vi "FTW-Actor-LocalMessage-Send.vi"(0 "FTW-ActorInstance In":refnum<class "FTW-ActorInstance.lvclass">, 5 "Message Header":string, 7 "Message Body":string, 11 "error in":errorcluster) -> (15 "error out":errorcluster)   [LabVIEW 2013, in "FTW-ActorInstance.lvclass"]
uses:
  FTW-ActorInstance.lvclass
  Message/Base/FTW-Message.lvclass
  FTW-ActorInstance.lvclass/FTW-ActorInstance.ctl
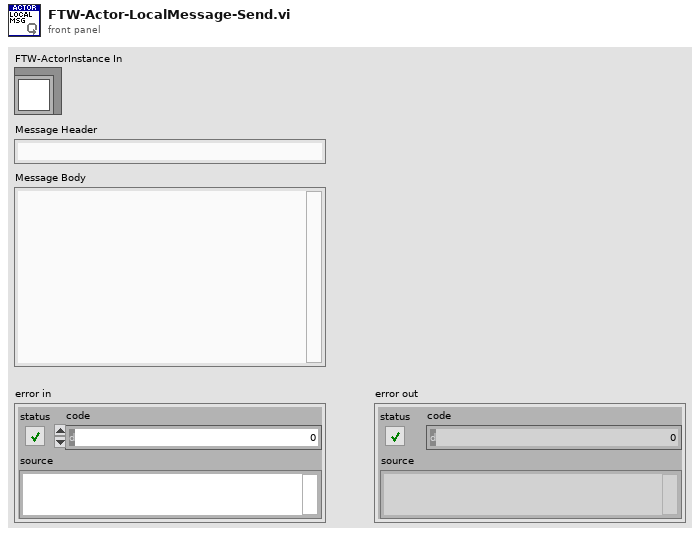
[diagram p1: front panel]
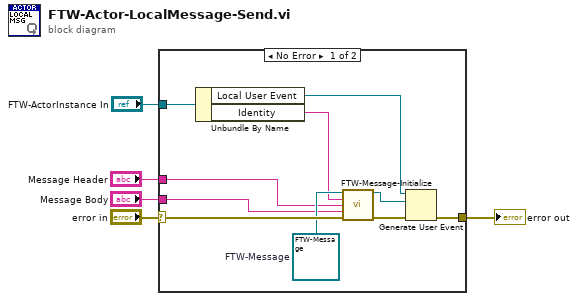
[diagram p0: block diagram]
diagram:
  n1 = case shown="No Error" "error in" {
    selector: "error in" -> [w12 w16]
    tunnel: "FTW-ActorInstance In" -> [w13 _]
    tunnel: [w11 w16] -> w3
    tunnel: "Message Header" -> [w7 _]
    tunnel: "Message Body" -> [w6 _]
    frame No Error {
      w10 = refnum<class "FTW-Message.lvclass"> refnum  # FTW-Message
      n2 = Unbundle By Name(w13) -> ("Local User Event"=w9:refnum<user-event>, "Identity"=w8:string)
      n3 = call-dynamic "FTW-Message-Initialize.vi"("FTW Message"=w10, "Sender Identity"=w8, "Message Header"=w7, "Message Body"=w6, "error in"=w12) -> ("FTW Message out"=w14:refnum<class "FTW-Message.lvclass">, "error out"=w15:errorcluster)  [unwired: 9 in]
      n4 = Generate User Event(user event=w9, event data cluster=w14, error in=w15) -> (error out=w11:errorcluster)  [unwired: 1 in, 1 out]
    }
    frame Error {
    }
  }
  "error out" <- w3
